vi "Agilis-standalone.vi"() -> ()   [LabVIEW 2011]
uses:
  <vilib>/Instr/_visa.llb/VISA Configure Serial Port (Instr).vi
panel:
  out "output p":dbl
  out "output °":dbl
  in  "minPos":dbl=68.14
  in  "Laser [%]":dbl(slide) min=0.0 max=100.0 step=0.1 scale=0.1..100.0
  in  "stop":bool
  out "Ist [°]":dbl(slide) scale=0.0..45.0
  in  "Soll [°]":dbl(slide) scale=0.0..70.0
  out "error out":errorcluster
  in  "VISA resource name":refnum<visa-resource-name>
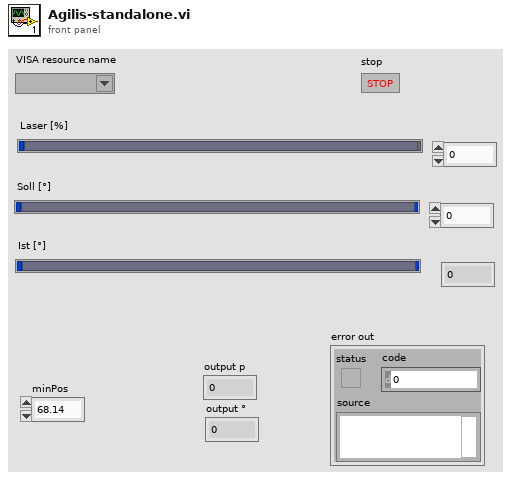
[diagram p1: front panel]
types:
  T1 = enum16{"NoOp", "GetStatus", "GetPosition", "SetPosition", "SetRelative", "GetError", "WriteRawAndRead", "clear", "switchOn"}
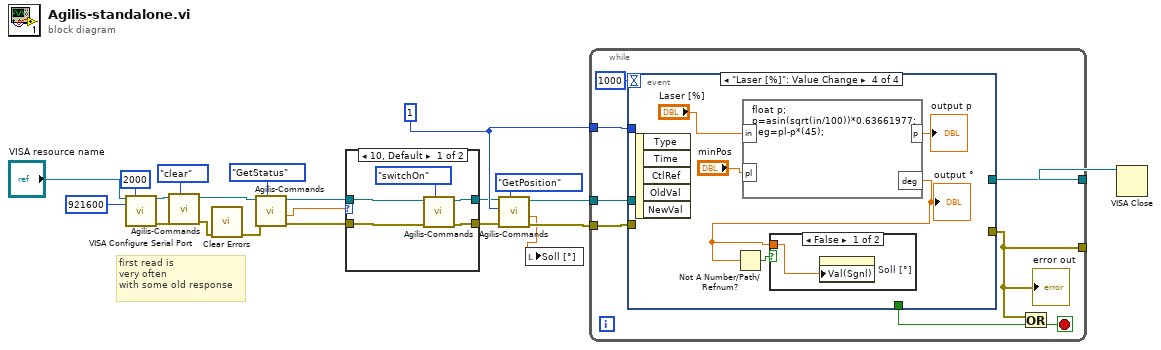
[diagram p0: block diagram]
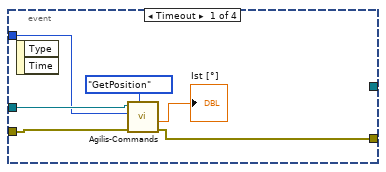
[diagram p3: hidden frame]
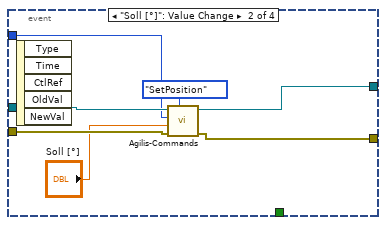
[diagram p4: hidden frame]
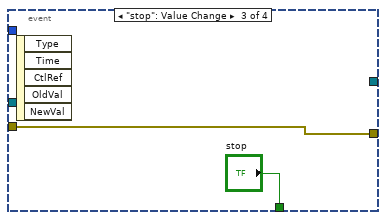
[diagram p5: hidden frame]
diagram:
  w12 = u8 1 ("Axis")
  # "first read is\nvery often \nwith some old response"
  n1 = call-poly "VISA Configure Serial Port"("VISA resource name"="VISA resource name", "timeout (10sec)"=u32 2000, "baud rate (9600)"=u32 921600) -> ("VISA resource name out"=w13:refnum<visa-resource-name>, "error out"=w14:errorcluster)  [unwired: 11 in]
  n2 = call "Agilis-Commands.vi"("Command in"=T1."clear", "error in (no error)"=w14, "VISA Refnum in"=w13) -> ("error out"=w10:errorcluster, "VISA resource name out"=w11:refnum<visa-resource-name>)  [unwired: 5 in, 2 out]
  n3 = call <vilib>:"Clear Errors.vi"("error in (no error)"=w10) -> ("error out"=w9:errorcluster)  [unwired: 6 in]
  n4 = call "Agilis-Commands.vi"("Command in"=T1."GetStatus", "error in (no error)"=w9, "VISA Refnum in"=w11) -> ("error out"=w7:errorcluster, "value"=w8:dbl, "VISA resource name out"=w5:refnum<visa-resource-name>)  [unwired: 5 in, 1 out]
  n5 = case shown="10, Default" w8 {
    tunnel: w7 -> [w26 w28]
    tunnel: [w25 w28] -> w6
    tunnel: w5 -> [w24 w27]
    tunnel: [w23 w27] -> w4
    frame 10, Default {
      n6 = call "Agilis-Commands.vi"("Command in"=T1."switchOn", "error in (no error)"=w26, "VISA Refnum in"=w24) -> ("error out"=w25:errorcluster, "VISA resource name out"=w23:refnum<visa-resource-name>)  [unwired: 5 in, 2 out]
    }
    frame 51 {
      # "OK"
    }
  }
  n7 = call "Agilis-Commands.vi"("Command in"=T1."GetPosition", "error in (no error)"=w6, "Axis in"=w12, "VISA Refnum in"=w4) -> ("error out"=w17:errorcluster, "value"=w16:dbl, "VISA resource name out"=w18:refnum<visa-resource-name>)  [unwired: 4 in, 1 out]
  n8 = local write "Soll [°]"(w16) -> ()
  n9 = while {
    tunnel: w18 -> [w35]
    tunnel: w17 -> [w34]
    tunnel: [w29] -> _
    tunnel: w12 -> [w33]
    tunnel: [w31] -> w15
    stop <- w30 stop-if-true
    n10 = event shown="[3] \"Laser [%]\": Value Change" {
      selector: _ -> [_ _ _ _]
      dyn-events: _ -> [_ _ _ _]
      timeout: 1000 -> [_ _ _ _]
      tunnel: w35 -> [w42 w49 _ _]
      tunnel: w34 -> [w40 w48 w50 _]
      tunnel: [w39 w47 w50 _] -> w29
      tunnel: w33 -> [w38 w46 _ _]
      tunnel: [_ _ "stop" _] -> w32
      tunnel: [_ w44 _ _] -> w31
      event Timeout {
        n11 = event-data() -> ()  [unwired: 1 in, 2 out]
        n12 = call "Agilis-Commands.vi"("Command in"=T1."GetPosition", "error in (no error)"=w40, "Axis in"=w38, "VISA Refnum in"=w42) -> ("error out"=w39:errorcluster, "value"=→"Ist [°]":dbl)  [unwired: 4 in, 2 out]
      }
      event "Soll [°]": Value Change {
        n13 = event-data() -> ()  [unwired: 1 in, 5 out]
        n14 = call "Agilis-Commands.vi"("Command in"=T1."SetPosition", "error in (no error)"=w48, "Value"="Soll [°]", "Axis in"=w46, "VISA Refnum in"=w49) -> ("error out"=w47:errorcluster, "VISA resource name out"=w44:refnum<visa-resource-name>)  [unwired: 3 in, 2 out]
      }
      event "stop": Value Change {
        n15 = event-data() -> ()  [unwired: 1 in, 5 out]
      }
      event "Laser [%]": Value Change {
        n16 = event-data() -> ()  [unwired: 1 in, 5 out]
        n17 = formula code="float p;\np=asin(sqrt(in/100))*0.63661977;\ndeg=pl-p*(45);"("in"="Laser [%]", "pl"="minPos") -> ("deg"=w52:dbl, "p"=→"output p":dbl)
        "output °" <- w52
        n18 = Not A Number/Path/Refnum?(number/path/refnum=w52) -> (NaN/Path/Refnum?=w53:bool)
        n19 = case shown="False" w53 {
          tunnel: w52 -> [w57 _]
          frame False {
            n20 = property on="Soll [°]" class="Slide (strict)"("Val(Sgnl)"=w57) -> ()  [unwired: 2 in, 2 out]
          }
          frame True {
          }
        }
      }
    }
    "error out" <- w29
    n21 = Or(x=w29, y=w32) -> (x .or. y?=w30:bool)
  }
  n22 = VISA Close(VISA resource name=w15) -> ()  [unwired: 1 in, 1 out]
